vi "DSF.Engine.Plugin.Get Transfer Group.vi"(10 "transfer group id":i32, 11 "Plugin in":refnum<class "DSF.Engine.Plugin.lvclass">) -> (2 "Transfer Group":refnum<class "DSF.Engine.Transfer Group.lvclass">, 3 "Plugin out":refnum<class "DSF.Engine.Plugin.lvclass">)   [LabVIEW 2017, in "DSF.Engine.lvlib" / "DSF.Engine.Plugin.lvclass"]
uses:
  DSF.Engine.Plugin.lvclass
  Transfer/DSF.Engine.Transfer Group.lvclass
  DSF.Engine.Plugin.lvclass/DSF.Engine.Plugin.ctl
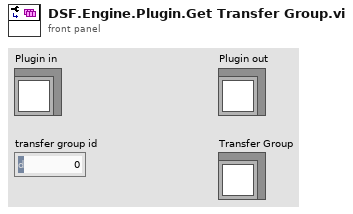
[diagram p1: front panel]
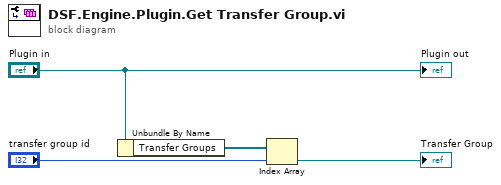
[diagram p0: block diagram]
diagram:
  n1 = Unbundle By Name("Plugin in") -> ("Transfer Groups"=w3:refnum<class "DSF.Engine.Transfer Group.lvclass">[])
  n2 = Index Array(array=w3, index="transfer group id") -> (element=→"Transfer Group":refnum<class "DSF.Engine.Transfer Group.lvclass">)
  "Plugin out" <- "Plugin in"
